vi "StreamEngine.Main.Stream.Start.vi"(7 "Stream.Qs.SubProcesses":T1, 8 "error in (no error)":errorcluster, 11 "Parameters":variant) -> (0 "error out":errorcluster, 2 "Stream Ref":T2, 3 "gRPC ID out":T2)   [LabVIEW 2025, in "XNET Bus Monitor Client.lvlib"]
uses:
  XNET Bus Monitor Client.lvlib
  <vilib>/gRPC/LabVIEW gRPC Library/Shared/grpcId.ctl
  Types/SubProcessEngine.QueueRefs.ctl
  Types/SubProcessEngine.CmdQueueData.ctl
  Types/SubProcessEngine.CmdQueueData.Cmd.ctl
  bus_monitor_client/RPC Messages/ni_bus_monitor_api_StreamBusRequest.ctl
  bus_monitor_client/RPC Messages/ni_bus_monitor_api_Session.ctl
  Types/StreamEngine.CmdQueueData.InitialSettings.ctl
  bus_monitor_client/bus_monitor_client.lvlib
  <vilib>/gRPC/LabVIEW gRPC Library/grpc-lvsupport-release.lvlib
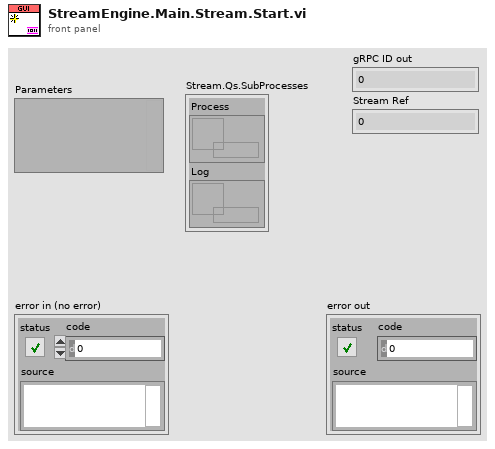
[diagram p1: front panel]
types:
  T1 = typedef "XNET Bus Monitor Client.lvlib/SubProcessEngine.QueueRefs.ctl" = cluster{"Process":refnum<queue>, "Log":refnum<queue>}
  T2 = typedef "grpc-lvsupport-release.lvlib/grpcId.ctl" = u64
  T3 = typedef "bus_monitor_client.lvlib/ni_bus_monitor_api_StreamBusRequest.ctl" = cluster{"session":T4}
  T4 = typedef "bus_monitor_client.lvlib/ni_bus_monitor_api_Session.ctl" = cluster{"name":string, "session_uid":string}
  T5 = typedef "XNET Bus Monitor Client.lvlib/StreamEngine.CmdQueueData.InitialSettings.ctl" = cluster{"gRPC ID":T2, "Session":T4, "Project Folder":path}
  T6 = typedef "XNET Bus Monitor Client.lvlib/SubProcessEngine.CmdQueueData.ctl" = cluster{"Cmd":T7, "Parameters":variant}
  T7 = typedef "XNET Bus Monitor Client.lvlib/SubProcessEngine.CmdQueueData.Cmd.ctl" = enum16{"Arm", "Publish", "Stop", "Exit"}
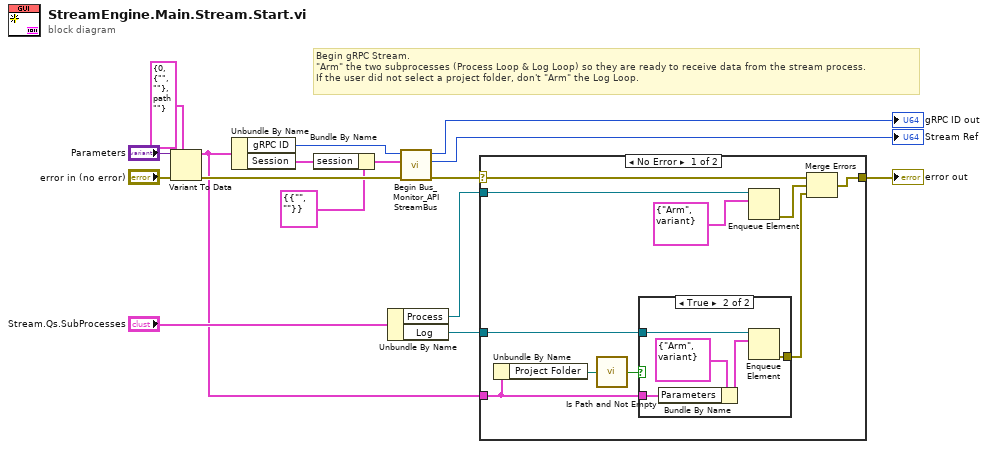
[diagram p0: block diagram]
diagram:
  # "Begin gRPC Stream.\n\"Arm\" the two subprocesses (Process Loop & Log Loop) so they are ready to receive data from the stream process.\nIf the user did not select a project folder, don't \"Arm\" the Log Loop."
  n1 = Variant To Data(error in="error in (no error)", type=T5 {"gRPC ID"=0, "Session"={"name"="", "session_uid"=""}, "Project Folder"=path ""} ("cluster"), Variant="Parameters") -> (data=w4:T5, error out=w10:errorcluster)
  n2 = Unbundle By Name(w4) -> ("gRPC ID"=w12:T2, "Session"=w1:T4)
  n3 = Bundle By Name(cluster=T3 {"session"={"name"="", "session_uid"=""}} ("Request Data"), "session"=w1) -> (w2:T3)
  n4 = Unbundle By Name("Stream.Qs.SubProcesses") -> ("Process"=w6:refnum<queue>, "Log"=w5:refnum<queue>)
  n5 = call "Begin Bus_Monitor_API StreamBus.vi"("error in"=w10, "Request Data"=w2, "gRPC ID"=w12) -> ("error out"=w9:errorcluster, "Call Id Out"=→"Stream Ref":T2, "gRPC ID out"=→"gRPC ID out":T2)  [unwired: 6 in]
  n6 = case shown="No Error" w9 {
    selector: w9 -> [w26 w32]
    tunnel: [w22 w32] -> w8
    tunnel: w6 -> [w25 _]
    tunnel: w5 -> [w24 _]
    tunnel: w4 -> [w19 _]
    frame No Error {
      n7 = Unbundle By Name(w19) -> ("Project Folder"=w18:path)
      n8 = call <vilib>:"Is Path and Not Empty.vi"("path"=w18) -> ("Is Path and Not Empty?"=w17:bool)  [unwired: 4 in]
      n9 = case shown="True" w17 {
        tunnel: w24 -> [_ w31]
        tunnel: [_ w29] -> w20
        tunnel: w19 -> [_ w28]
        frame False {
        }
        frame True {
          n10 = Bundle By Name(cluster=T6 {"Cmd"=enum."Arm", "Parameters"=variant} ("element"), "Parameters"=w28) -> (w30:T6)
          n11 = Enqueue Element(queue=w31, element=w30) -> (error out=w29:errorcluster)  [unwired: 2 in, 2 out]
        }
      }
      n12 = Enqueue Element(queue=w25, element=T6 {"Cmd"=enum."Arm", "Parameters"=variant}) -> (error out=w21:errorcluster)  [unwired: 2 in, 2 out]
      n13 = Merge Errors(w26, w21, w20) -> (w22:errorcluster)
    }
    frame Error {
    }
  }
  "error out" <- w8
